vi "Move Window Into Unused Position.vi"(10 "VI in":refnum<vi>, 11 "set in":set{T1}(c389)) -> (2 "VI out":refnum<vi>, 3 "set out":set{T1}(c389))   [LabVIEW 2023]
uses:
  <vilib>/Utility/miscctls.llb/LVRectTypeDef.ctl
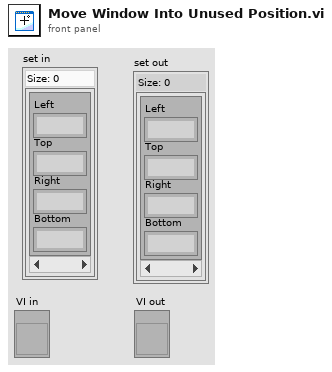
[diagram p1: front panel]
types:
  T1 = typedef "LVRectTypeDef.ctl" = cluster{"Left":i16, "Top":i16, "Right":i16, "Bottom":i16}
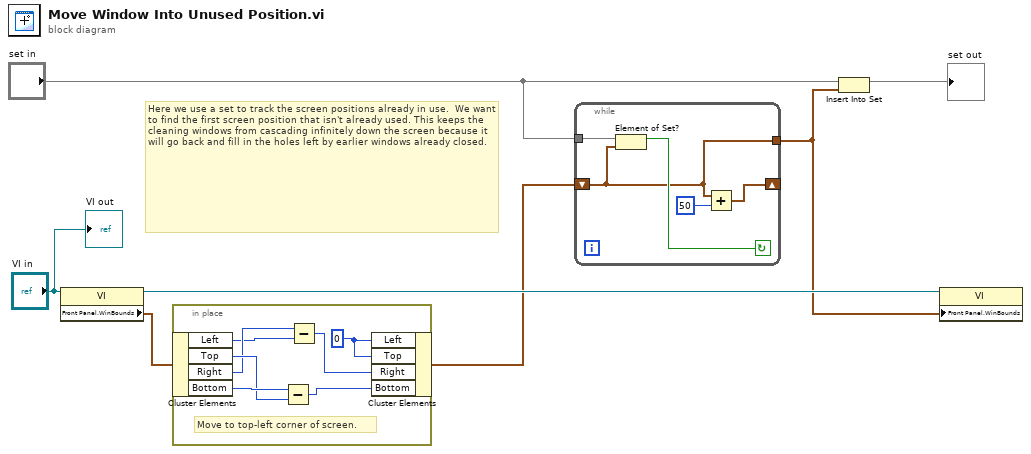
[diagram p0: block diagram]
diagram:
  # "Here we use a set to track the screen positions already in use.  We want to find the first screen position that isn't already used. This keeps the cleaning windows from cascading infinitely down the screen because it will go back and fill in the holes left by earlier windows already closed."
  n1 = property class="VI"(reference="VI in") -> (reference out=w7:refnum<vi>, "Front Panel.WinBounds"=w6:T1)  [unwired: 1 in, 1 out]
  n2 = in-place {
    w8 = i16 0 ("Left")
    # "Move to top-left corner of screen."
    n3 = in-place-cluster #1(w6) -> ("Left"=w9:i16, "Top"=w13:i16, "Right"=w10:i16, "Bottom"=w14:i16)
    n4 = Subtract(x=w14, y=w13) -> (x-y=w12:i16)
    n5 = Subtract(x=w10, y=w9) -> (x-y=w11:i16)
    n6 = in-place-cluster #1("Left"=w8, "Top"=w8, "Right"=w11, "Bottom"=w12) -> (w5:T1)
  }
  n7 = while {
    tunnel: "set in" -> [w19]
    shift-right: [w16] -> _
    shift-left: w5 -> [w15]
    tunnel: [w15] -> w3
    stop <- w18 continue-if-true
    n8 = Element of Set?(10:w15, 11:w19) -> (3:w18:bool)
    n9 = Add(x=w15, y=i16 50 ("Left")) -> (x+y=w16:T1)
  }
  n10 = Insert Into Set(10:w3, 11:"set in") -> (3:→"set out":set{T1})  [unwired: 1 out]
  n11 = property class="VI"(reference=w7, "Front Panel.WinBounds"=w3) -> ()  [unwired: 1 in, 2 out]
  "VI out" <- "VI in"
